vi "AdjustMagnetDiscTiming.vi"(1 "Input Trigger Data":T3) -> (0 "Output Trigger Data":T3)   [LabVIEW 2016]
uses:
  Ctrl_Signal.ctl
  Ctrl_Signal_Map.ctl
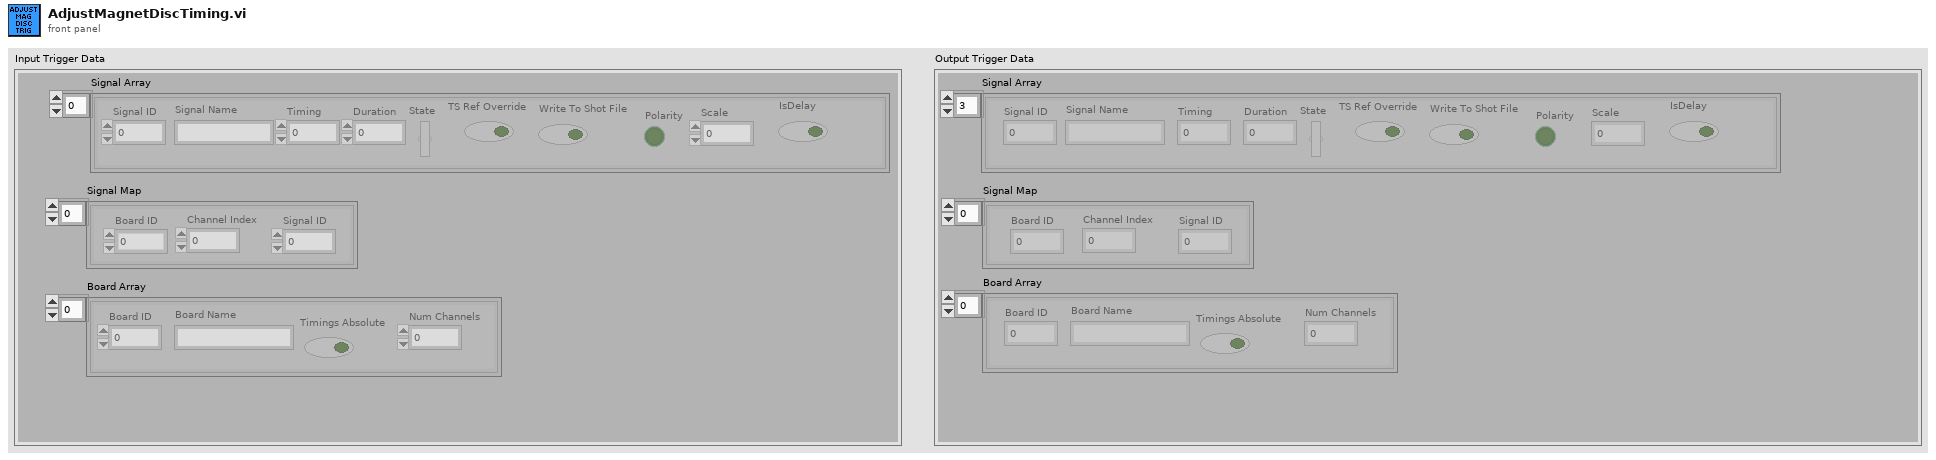
[diagram p1: front panel]
types:
  T1 = typedef "Ctrl_Signal.ctl" = cluster{"Signal Name":string, "Timing":dbl, "Duration":dbl, "State":bool, "TS Ref Override":bool, "Write To Shot File":bool, "Polarity":bool, "Signal ID":dbl, "Scale":dbl, "IsDelay":bool}
  T2 = typedef "Ctrl_Signal_Map.ctl" = cluster{"Channel Index":dbl, "Board ID":dbl, "Signal ID":dbl}
  T3 = cluster{"Signal Array":T1[], "Signal Map":T2[], "Board Array":cluster{"Board ID":dbl, "Board Name":string, "Timings Absolute":bool, "Num Channels":dbl}[]}
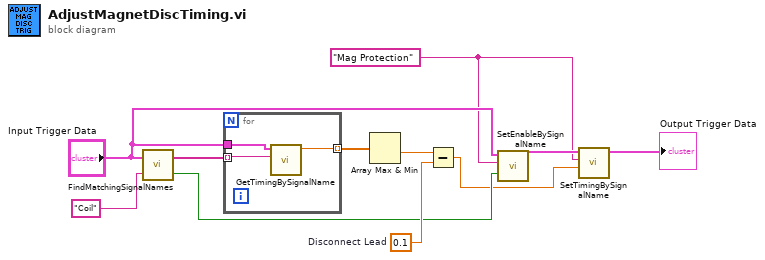
[diagram p0: block diagram]
diagram:
  w7 = 0.1  # Disconnect Lead
  w3 = "Mag Protection"
  n1 = call "FindMatchingSignalNames.vi"("Signal Name"="Coil", "Trigger Data"="Input Trigger Data") -> ("Anything Found"=w5:bool, "Signal Names Matched"=w10:string[])
  n2 = for {
    tunnel: w10 -> [w14] mode=indexing
    tunnel: "Input Trigger Data" -> [w13]
    tunnel: [w12] -> w9 mode=indexing
    n3 = call "GetTimingBySignalName.vi"("Signal Name"=w14, "Trigger Data"=w13) -> ("Timing"=w12:dbl)  [unwired: 9 in]
  }
  n4 = Array Max & Min(array=w9) -> (min value=w8:dbl)  [unwired: 3 out]
  n5 = Subtract(x=w8, y=w7) -> (x-y=w2:dbl)
  n6 = call "SetEnableBySignalName.vi"("State"=w5, "Signal Name"=w3, "Trigger Data Input"="Input Trigger Data") -> ("Trigger Data Output"=w4:T3)  [unwired: 8 in]
  n7 = call "SetTimingBySignalName.vi"("Timing"=w2, "Signal Name"=w3, "Trigger Data Input"=w4) -> ("Trigger Data Output"=→"Output Trigger Data":T3)  [unwired: 8 in]
